vi "FindInstrument_libESP301.vi"(6 "search string/char ()":string, 8 "error in (no error)":errorcluster) -> (0 "error out":errorcluster, 1 "Found Interface Names":string[](array[string]), 2 "Found Resource Names":string[](array[string]))   [LabVIEW 2018, in "Newport ESP301.lvlib"]
doc: "Query the Instruments in the system.\n\nFinds and connects through VISA.\n\nsearch string:\nSearch string can be used to filter results to a particular type that has search string in it Interface Name. It is optional and blank by default.\n\nOutput Found Resource Names are VISA Resource names and Found Interface Names are the matching Interface names."
uses:
  Newport ESP301.lvlib
  <vilib>/Instr/_visa.llb/VISA Find Search Mode.ctl
panel:
  # "Newport Find Instruments"
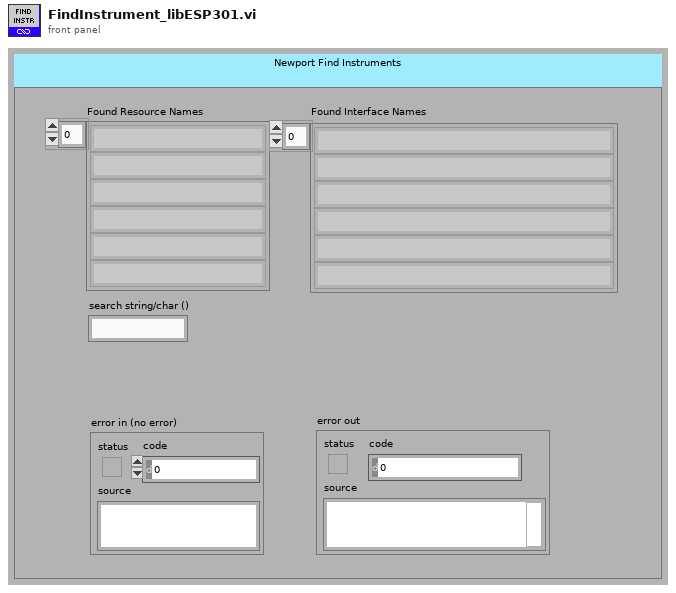
[diagram p1: front panel]
types:
  T1 = typedef "VISA Find Search Mode.ctl" = u32
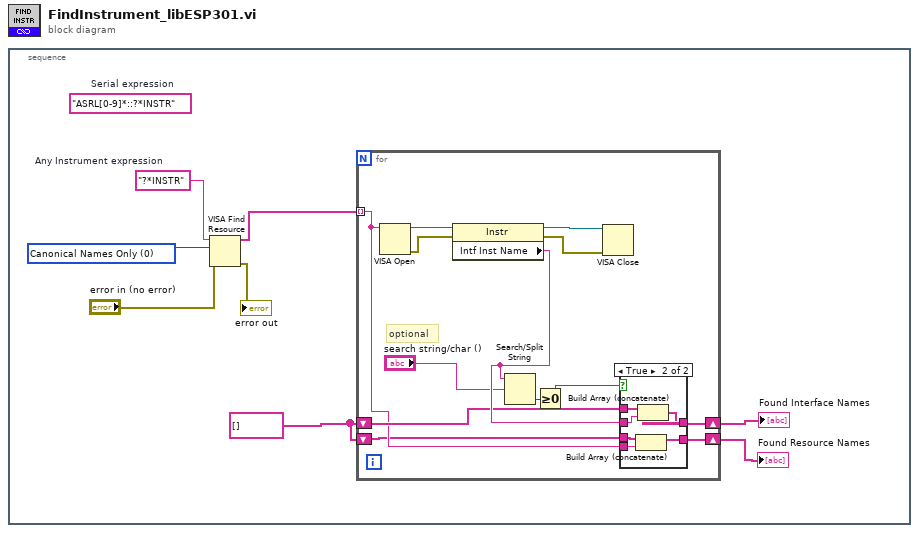
[diagram p0: block diagram]
diagram:
  n1 = stacked-sequence {
    frame #0 {
      (unwired) "ASRL[0-9]*::?*INSTR"  # Serial expression
      w3 = string[] [] ("Array 2")
      w4 = T1 0 items=["Canonical Names Only"=0, "Aliases Only"=2, "Include Matching Aliases"=3, "Include All Aliases"=4] ("Search Mode")
      w5 = "?*INSTR"  # Any Instrument expression
      n2 = VISA Find Resource(8:"error in (no error)", 10:w4, 11:w5) -> (0:→"error out":errorcluster, 3:w7:string[])  [unwired: 1 out]
      n3 = for {
        tunnel: w7 -> [w12] mode=indexing
        shift-right: [w15] -> w6
        shift-left: w3 -> [w13]
        shift-right: [w10] -> w2
        shift-left: w3 -> [w11]
        # "optional"
        n4 = VISA Open(VISA resource name=w12) -> (VISA resource name=w21:refnum<visa-resource-name>, error out=w18:errorcluster)  [unwired: 4 in]
        n5 = property class="Instr"(reference=w21, error in=w18) -> (reference out=w20:refnum<visa-resource-name>, error out=w19:errorcluster, "Intf Inst Name"=w14:string)
        n6 = Search/Split String(string=w14, search string/char (-)="search string/char ()") -> (offset of match=w17:i32)  [unwired: 1 in, 2 out]
        n7 = Greater Or Equal To 0?(x=w17) -> (x >= 0?=w16:bool)
        n8 = VISA Close(VISA resource name=w20, error in (no error)=w19) -> ()  [unwired: 1 out]
        n9 = case shown="True" w16 {
          tunnel: w13 -> [w23 w28]
          tunnel: [w23 w29] -> w15
          tunnel: w14 -> [_ w27]
          tunnel: w12 -> [_ w26]
          tunnel: w11 -> [w22 w25]
          tunnel: [w22 w24] -> w10
          frame False {
          }
          frame True {
            n10 = Build Array (concatenate)(w25, w26) -> (w24:string[])
            n11 = Build Array (concatenate)(w28, w27) -> (w29:string[])
          }
        }
      }
      "Found Resource Names" <- w2
      "Found Interface Names" <- w6
    }
  }
